vi "Cryostation Monitor and Control.vi"() -> ()   [LabVIEW 2020, in "instrument.Cryostation.lvclass"]
doc: "This VI will launch the Cryostation Instrument backend that will contunously monitor the state of the instrument and log to PGSQL."
uses:
  instrument.Cryostation/instrument.Cryostation.lvclass
  <userlib>/_OpenG.lib/appcontrol/appcontrol.llb/openg_application_control.lvlib
  <vilib>/JKI/JKI SMO/SMO/SMO.lvclass
  <vilib>/JKI/JKI SMO/SMO/Typedefs/SMOState --Enum.ctl
  <vilib>/JKI/JKI SMO/SMO.UI/SMO.UI.lvclass
  <userlib>/LevyLab/Instrument Framework/Instrument UI/Instrument UI.lvclass
  <userlib>/LevyLab/Instrument Framework/Instrument/Instrument.lvclass
  instrument.Cryostation UI/Instrument UI.Cryostation.lvclass
  C:/Program Files (x86)/National Instruments/LabVIEW 2020/user.lib/LevyLab/Instrument Framework/Instrument Types/Cryostat/Instrument.Cryostat.lvclass
  C:/Program Files (x86)/National Instruments/LabVIEW 2020/user.lib/LevyLab/Instrument Framework/Instrument/Instrument.lvclass
  C:/Program Files (x86)/National Instruments/LabVIEW 2020/vi.lib/JKI/JKI SMO/SMO/SMO.lvclass
  D:/Montana-Instruments-Cryostation/lvsrc/instrument.Cryostation/instrument.Cryostation.lvclass
  C:/Program Files (x86)/National Instruments/LabVIEW 2020/user.lib/LevyLab/Instrument Framework/Instrument UI/Instrument UI.lvclass
  C:/Program Files (x86)/National Instruments/LabVIEW 2020/vi.lib/JKI/JKI SMO/SMO.UI/SMO.UI.lvclass
  D:/Montana-Instruments-Cryostation/lvsrc/instrument.Cryostation UI/Instrument UI.Cryostation.lvclass
panel:
  out "version":string
  in  "Examine Configuration.ini":bool
  in  "Debug Mode":bool
  in  "Stop Application":bool caption="Stop"
  in  "Start Application":bool caption="Play"
  in  "Splash Status":string="Push Start to Start..." caption="String"
  out "UI SMO State":T1=enum."Stopped"
  out "SMO State":T1
  out "error out":errorcluster
  # "PPMS Monitor and Control.vi"
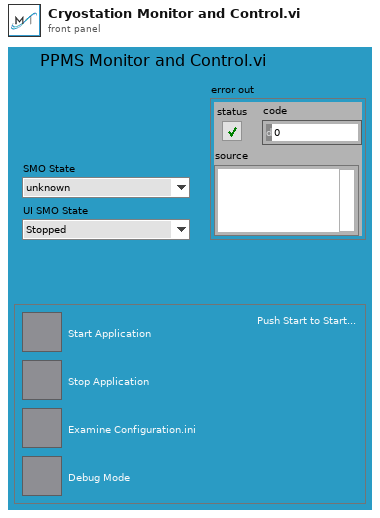
[diagram p1: front panel]
types:
  T1 = typedef "SMO.lvclass/SMOState --Enum.ctl" = enum16{"unknown", "Created", "Started", "Stopped"}
  T2 = enum32{"Invalid", "Standard", "Closed", "Hidden", "Minimized", "Maximized"}
  T3 = enum32{"invalid app kind", "Development System", "Run Time System", "Student Edition", "Embedded LabVIEW", "Evaluation", "Custom"}
  T4 = cluster{"Core":cluster{"Current VI Reference":refnum<vi>, "Close Panel on Exit?":bool}, "Instrument":refnum<class "instrument.Cryostation.lvclass">, "Instrument UI":refnum<class "Instrument UI.Cryostation.lvclass">}
  T5 = cluster{"Current VI Reference":refnum<vi>, "Close Panel on Exit?":bool}
  T6 = typedef "SMO.lvclass/Public Events.ctl" = cluster{"Error":refnum<user-event>, "State":refnum<user-event>, "Reserve State":refnum<user-event>}
  T7 = cluster{"Event Registration Refnum":refnum<event-registration>, "Event Registration Refnum":refnum<event-registration>}
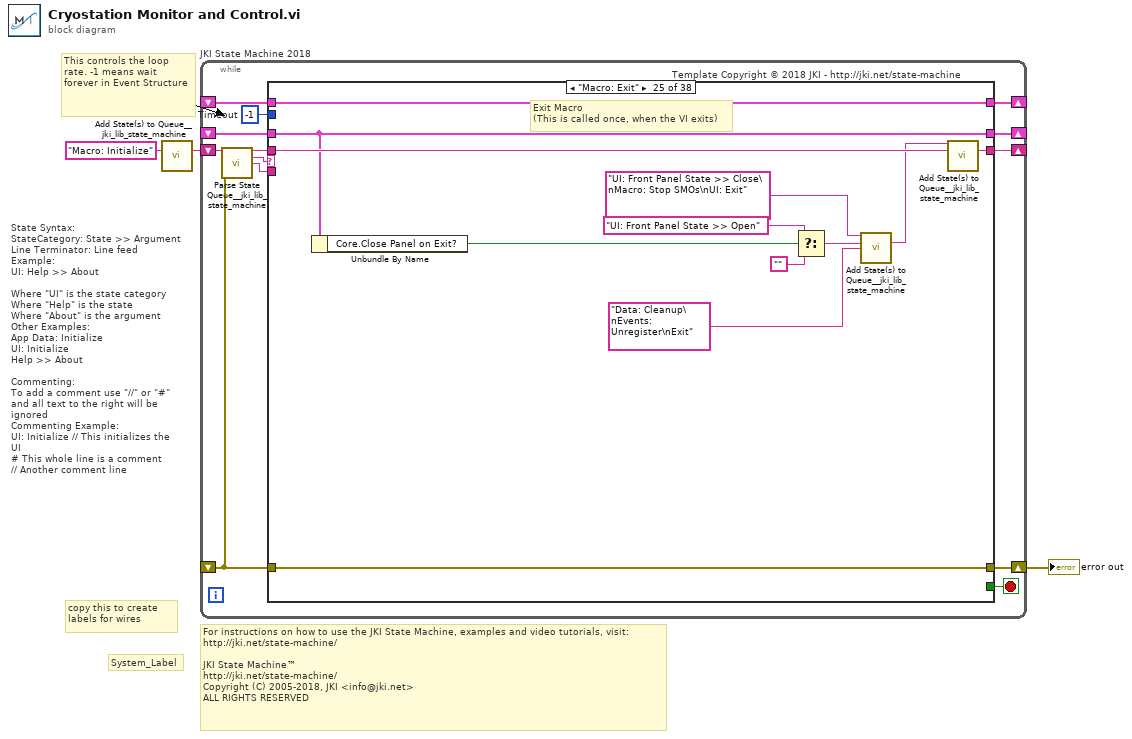
[diagram p0: block diagram]
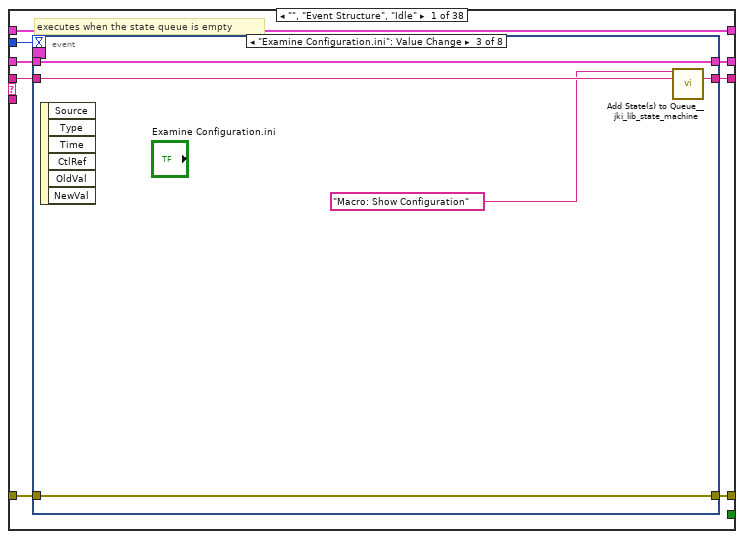
[diagram p2: hidden frame]
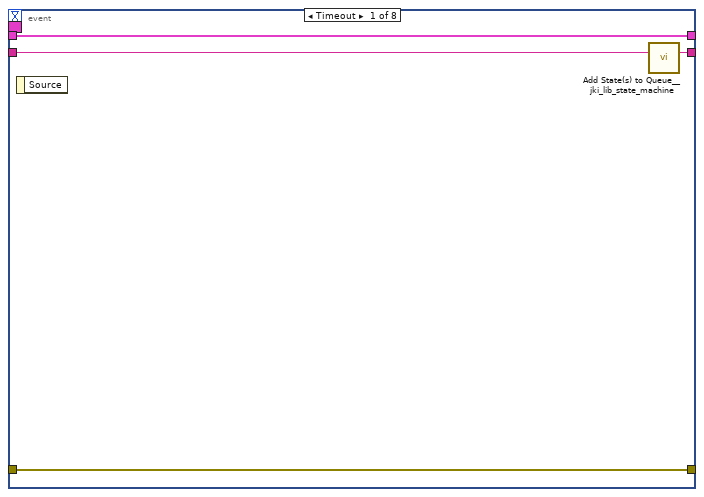
[diagram p3: hidden frame]
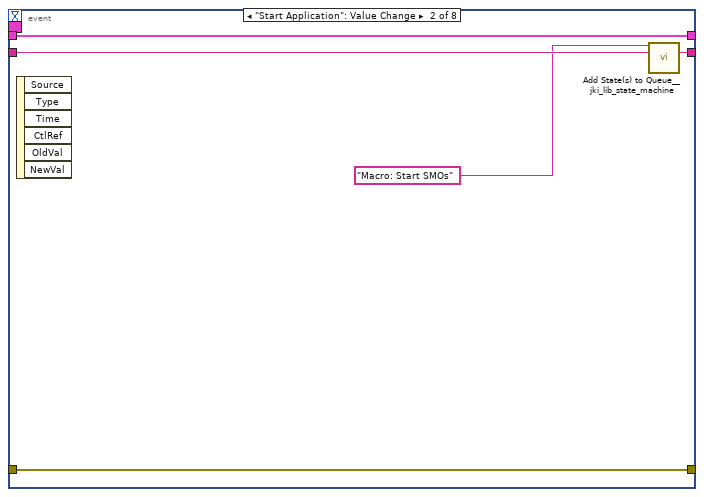
[diagram p4: hidden frame]
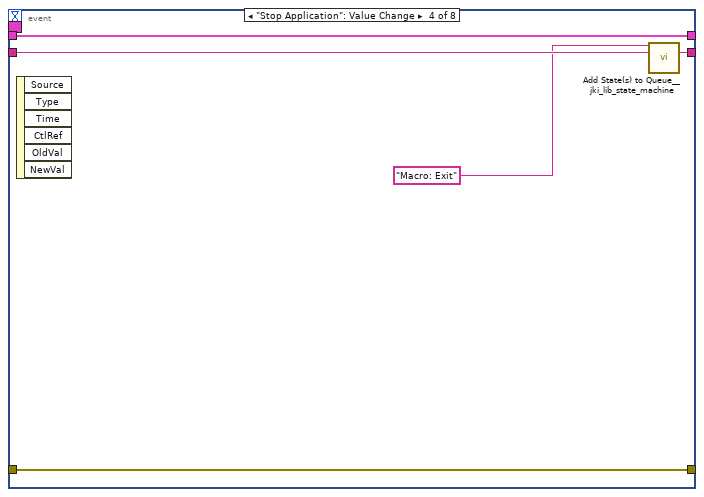
[diagram p5: hidden frame]
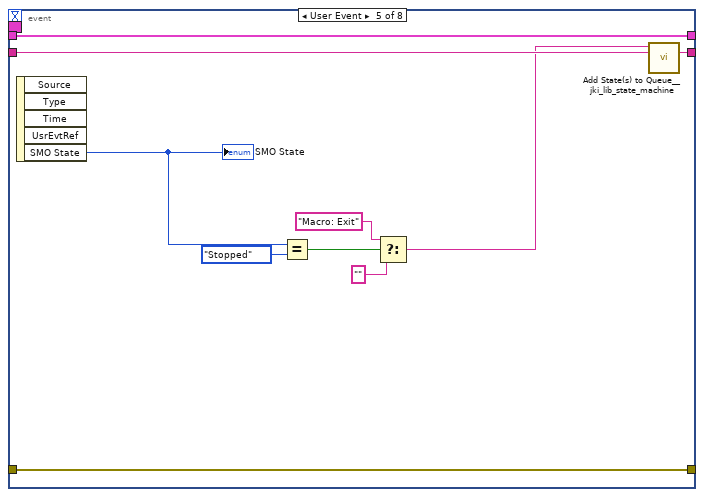
[diagram p6: hidden frame]
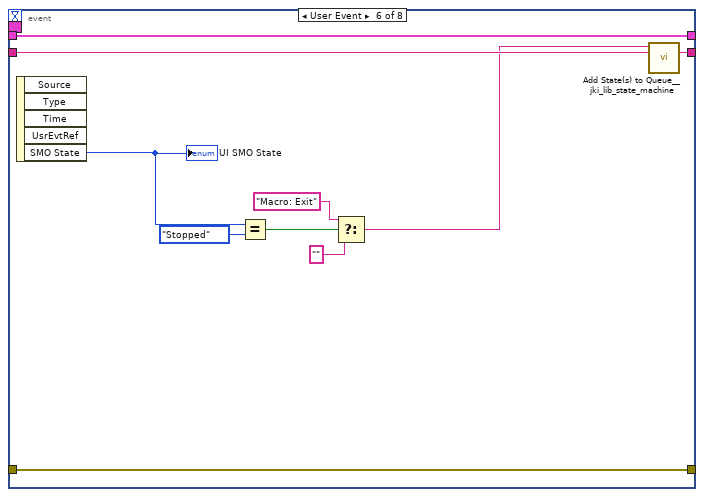
[diagram p7: hidden frame]
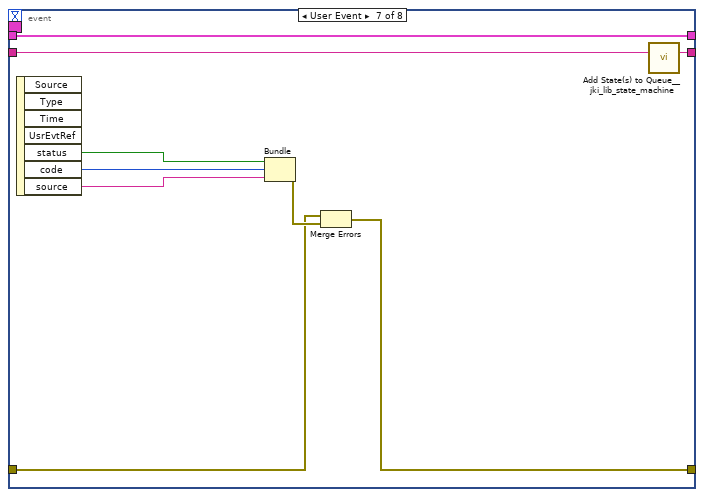
[diagram p8: hidden frame]
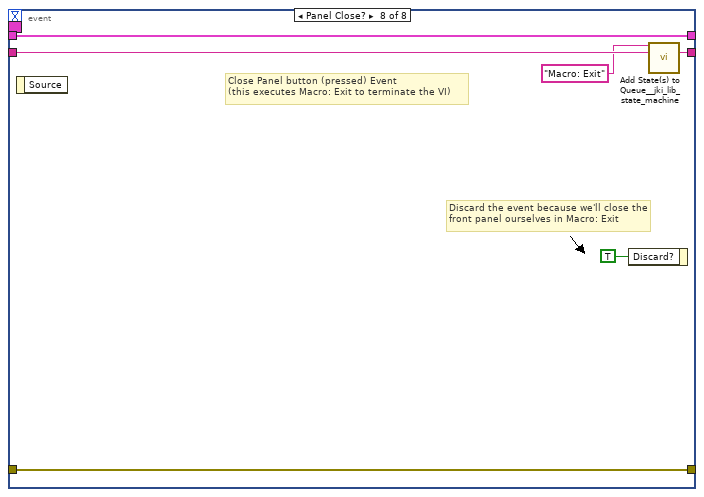
[diagram p9: hidden frame]
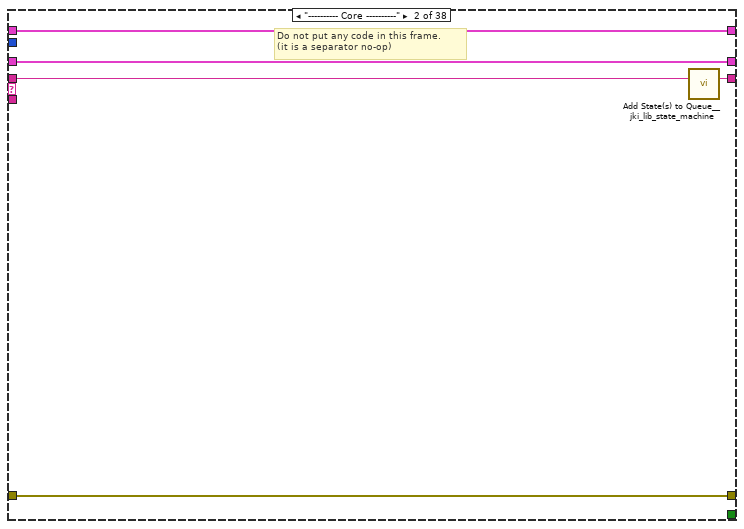
[diagram p10: hidden frame]
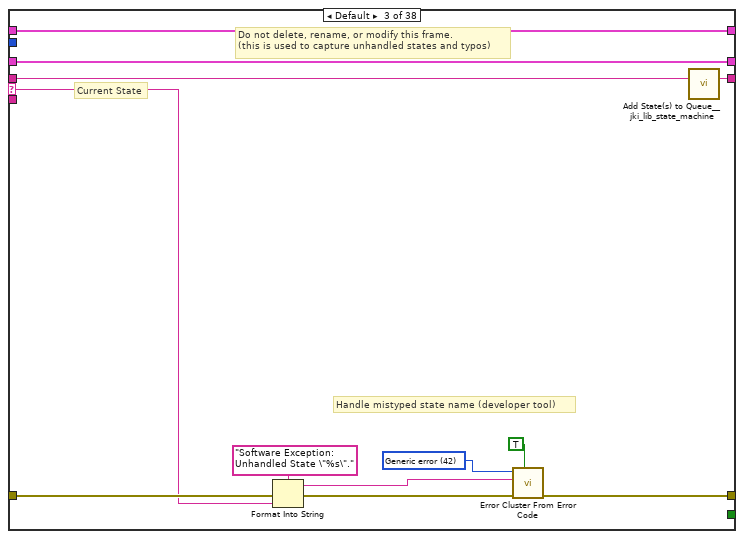
[diagram p11: hidden frame]
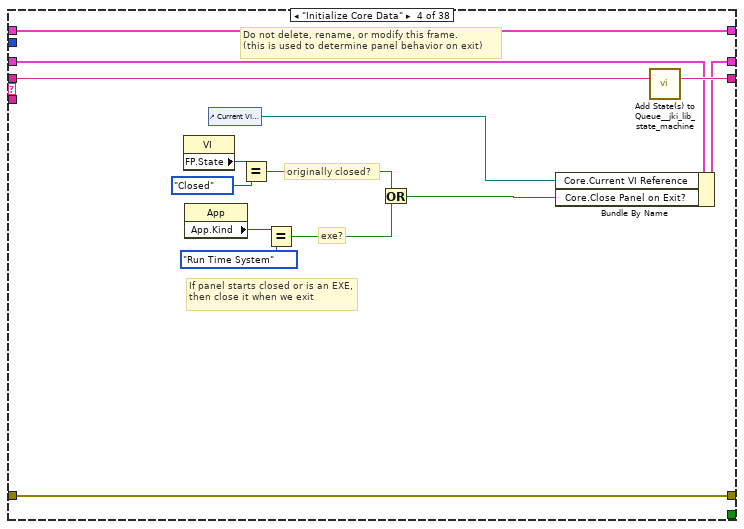
[diagram p12: hidden frame]
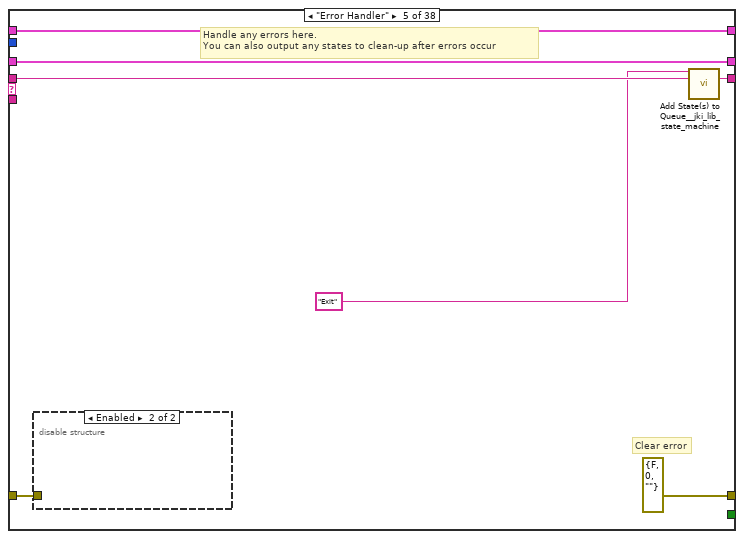
[diagram p13: hidden frame]
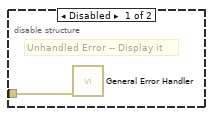
[diagram p14: hidden frame]
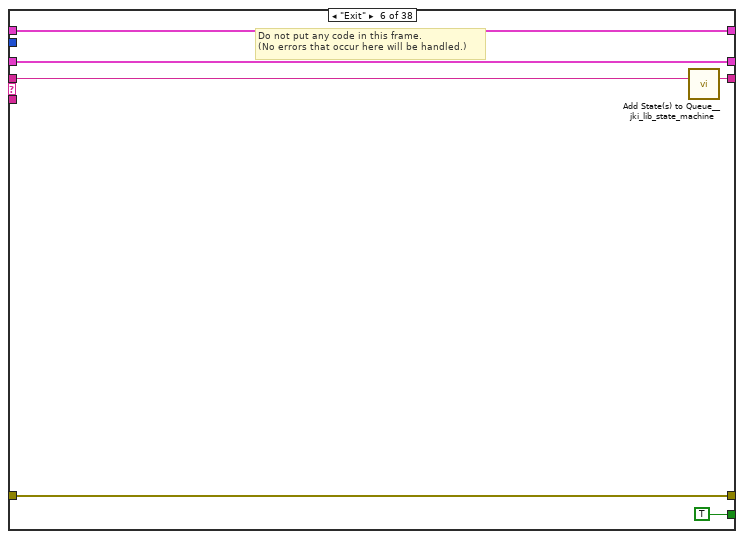
[diagram p15: hidden frame]
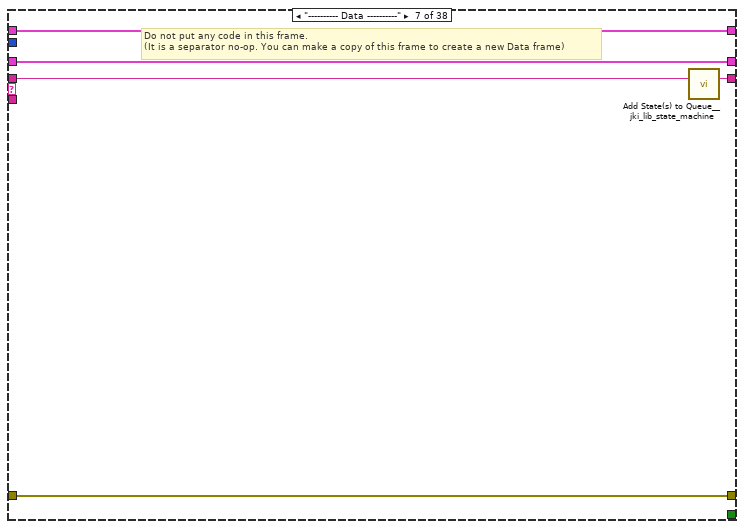
[diagram p16: hidden frame]
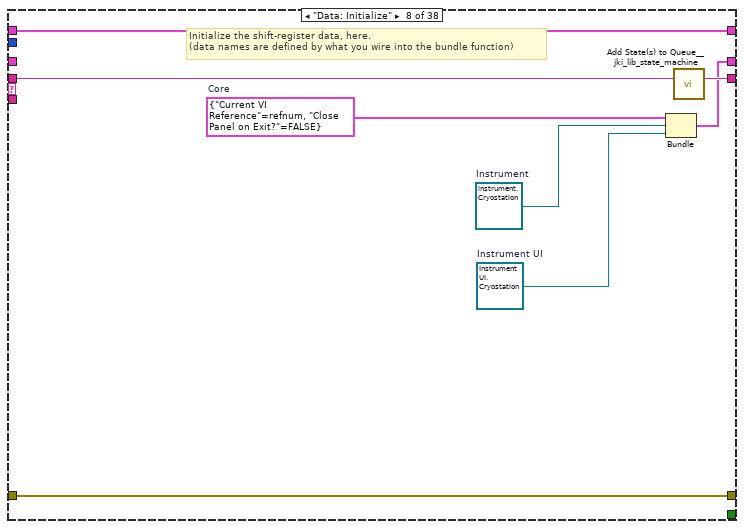
[diagram p17: hidden frame]
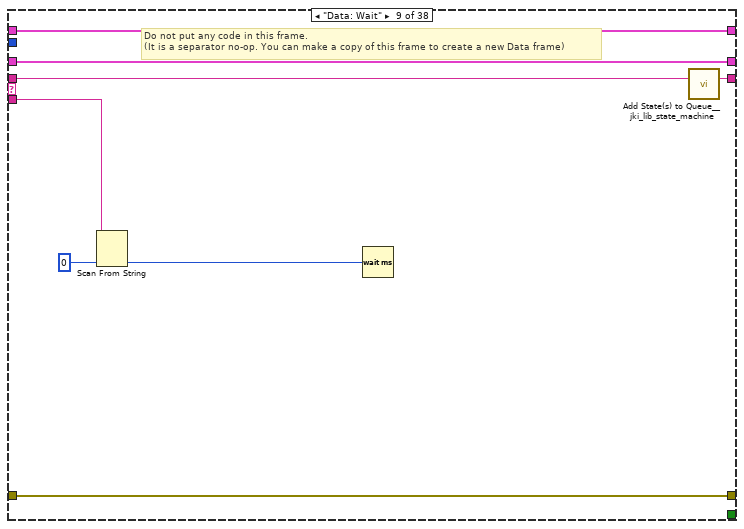
[diagram p18: hidden frame]
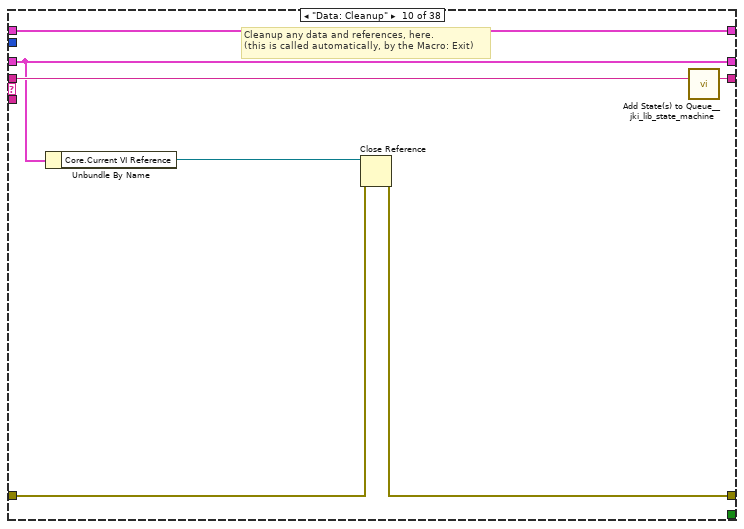
[diagram p19: hidden frame]
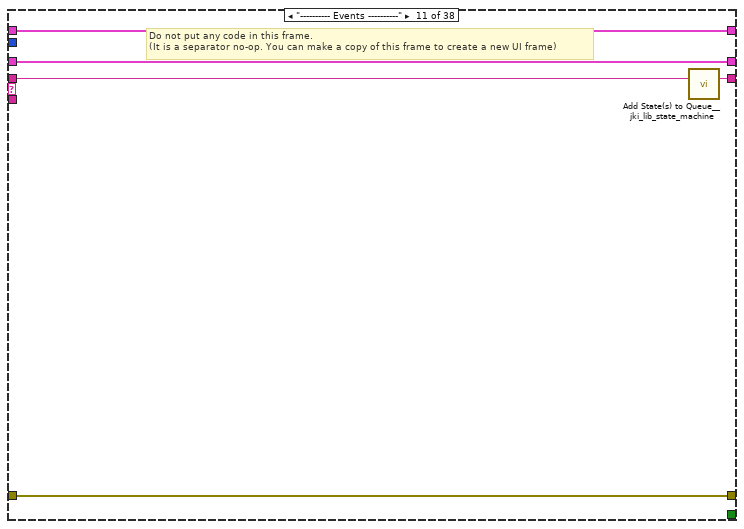
[diagram p20: hidden frame]
diagram:
  # "For instructions on how to use the JKI State Machine, examples and video tutorials, visit:\nhttp://jki.net/state-machine/\n\nJKI State Machine™\nhttp://jki.net/state-machine/\nCopyright (C) 2005-2018, JKI <info@jki.net>\nALL RIGHTS RESERVED"
  # "State Syntax:\nStateCategory: State >> Argument\nLine Terminator: Line feed\nExample:\nUI: Help >> About\n\nWhere \"UI\" is the state category\nWhere \"Help\" is the state\nWhere \"About\" is the argument\nOther Examples:\nApp Data: Initialize\nUI: Initialize\nHelp >> About\n\nCommenting:\nTo add a comment use \"//\" or \"#\" and all text to the right will be ignored\nCommenting Example:\nUI: Initialize // This initializes the UI\n# This whole line is a comment\n// Another comment line"
  # "copy this to create labels for wires"
  # "This controls the loop rate. -1 means wait forever in Event Structure"
  # "System_Label"
  n1 = call <vilib>:"Add State(s) to Queue__jki_lib_state_machine.vi"("State(s) in (\"\")"="Macro: Initialize") -> ("States Out"=w3:string)  [unwired: 14 in]
  n2 = while "JKI State Machine 2018" {
    shift-right: [w9] -> _
    shift-left: _ -> [w4]
    shift-right: [w12] -> w1
    shift-left: _ -> [w7]
    shift-right: [w11] -> _
    shift-left: w3 -> [w13]
    shift-right: [w6] -> _
    shift-left: _ -> [w5]
    stop <- w10 stop-if-true
    w8 = -1  # Timeout
    # "Template Copyright © 2018 JKI - http://jki.net/state-machine"
    n3 = call <vilib>:"Parse State Queue__jki_lib_state_machine.vi"("State Queue"=w13, "Error In (no error)"=w7) -> ("Remaining States"=w15:string, "Current State"=w16:string, "Arguments"=w14:string)  [unwired: 11 in]
    n4 = case shown="\"Macro: Exit\"" w16 {
      selector: w16 -> [_ _ w85 _ _ _ _ _ _ _ _ _ _ _ _ _ _ _ _ _ _ _ _ _ _ _ _ _ _ _ _ _ _ _ _ _ _ _]
      tunnel: w15 -> [w24 w83 w89 w109 w116 w123 w128 w136 w144 w151 w156 w169 w175 w180 w189 w196 w208 w282 w287 w292 w298 w304 w310 w316 w328 w333 w343 w352 w362 w369 w380 w395 w410 w425 w440 w449 w456 w461]
      tunnel: w14 -> [_ _ _ _ _ _ _ _ w137 _ _ _ _ _ _ w191 w202 _ _ _ _ _ _ _ _ _ _ _ _ _ _ _ _ _ _ _ w453 _]
      tunnel: [w21 w81 w91 w106 errorcluster {"status"=FALSE, "code"=0, "source"=""} ("error out") w120 w126 w133 w142 w147 w154 w158 w170 w178 w184 w192 w205 w278 w285 w290 w296 w302 w308 w314 w326 w331 w339 w344 w354 w363 w376 w391 w406 w422 w437 w447 w451 w459] -> w12
      tunnel: w7 -> [w20 w81 w90 w106 w112 w120 w126 w133 w142 w148 w154 w160 w171 w178 w186 w193 w206 w277 w285 w290 w296 w302 w308 w314 w326 w331 w340 w345 w355 w364 w373 w387 w403 w420 w433 w447 w452 w459]
      tunnel: [w23 w82 w88 w108 w115 w122 w127 w135 w143 w150 w155 w168 w174 w179 w188 w195 w207 w281 w286 w291 w297 w303 w309 w315 w327 w332 w342 w351 w361 w368 w379 w394 w409 w424 w439 w448 w455 w460] -> w11
      tunnel: [_ _ _ _ _ TRUE _ _ _ _ _ _ _ _ _ _ _ _ _ _ _ _ _ _ _ _ _ _ _ _ _ _ _ _ _ _ _ _] -> w10
      tunnel: [w19 w80 w87 w107 w113 w121 w125 w134 w141 w146 w153 w163 w173 w177 w187 w194 w204 w275 w284 w289 w295 w301 w307 w313 w325 w330 w338 w347 w356 w366 w377 w392 w407 w421 w436 w446 w454 w458] -> w9
      tunnel: w8 -> [w18 _ _ _ _ _ _ _ _ _ _ _ _ _ _ _ _ _ _ _ _ _ _ _ _ _ _ _ _ _ _ _ _ _ _ _ _ _]
      tunnel: [w17 w79 w84 w96 w110 w118 w124 w131 w140 w145 w152 w166 w172 w176 w185 w190 w201 w280 w283 w288 w293 w300 w306 w312 w319 w329 w341 w350 w360 w367 w378 w393 w408 w423 w438 w445 w450 w457] -> w6
      tunnel: w5 -> [w17 w79 w84 w96 w110 w118 w124 w131 w140 w145 w152 _ w172 w176 w185 w190 w201 w280 w283 w288 w293 w300 w306 w312 w319 w329 w341 w350 w360 w367 w378 w393 w408 w423 w438 w445 w450 w457]
      tunnel: w4 -> [w22 w80 w87 w102 w113 w121 w125 _ w141 w146 w153 w163 w173 w177 w187 w194 w204 w274 w284 w289 w295 w301 w307 w313 w325 w330 w335 w348 w357 w366 w377 w392 w407 w421 w436 w446 w454 w458]
      frame "", "Event Structure", "Idle" {
        # "executes when the state queue is empty"
        n5 = event shown="[2] \"Examine Configuration.ini\": Value Change" {
          selector: w17 -> [_ _ _ _ _ _ _ _]
          dyn-events: _ -> [_ _ _ _ _ _ _ _]
          timeout: w18 -> [_ _ _ _ _ _ _ _]
          tunnel: w24 -> [w28 w33 w38 w43 w53 w63 w72 w78]
          tunnel: [w27 w32 w37 w42 w52 w62 w71 w77] -> w23
          tunnel: w22 -> [w25 w30 w35 w40 w50 w60 w70 w75]
          tunnel: [w26 w31 w36 w41 w51 w61 w67 w76] -> w21
          tunnel: w20 -> [w26 w31 w36 w41 w51 w61 w68 w76]
          tunnel: [w25 w30 w35 w40 w50 w60 w70 w75] -> w19
          event Timeout {
            n6 = event-data() -> ()  [unwired: 1 in, 1 out]
            n7 = call <vilib>:"Add State(s) to Queue__jki_lib_state_machine.vi"("State(s) in (\"\")"=w28) -> ("States Out"=w27:string)  [unwired: 14 in]
          }
          event "Start Application": Value Change {
            n8 = event-data() -> ()  [unwired: 1 in, 6 out]
            n9 = call <vilib>:"Add State(s) to Queue__jki_lib_state_machine.vi"("State(s) in Front (\"\")"="Macro: Start SMOs" ("State(s) in Front (\"\")"), "State(s) in (\"\")"=w33) -> ("States Out"=w32:string)  [unwired: 13 in]
          }
          event "Examine Configuration.ini": Value Change {
            n10 = event-data() -> ()  [unwired: 1 in, 6 out]
            n11 = call <vilib>:"Add State(s) to Queue__jki_lib_state_machine.vi"("State(s) in Front (\"\")"="Macro: Show Configuration" ("State(s) in Front (\"\")"), "State(s) in (\"\")"=w38) -> ("States Out"=w37:string)  [unwired: 13 in]
          }
          event "Stop Application": Value Change {
            n12 = event-data() -> ()  [unwired: 1 in, 6 out]
            n13 = call <vilib>:"Add State(s) to Queue__jki_lib_state_machine.vi"("State(s) in Front (\"\")"="Macro: Exit" ("State(s) in Front (\"\")"), "State(s) in (\"\")"=w43) -> ("States Out"=w42:string)  [unwired: 13 in]
          }
          event User Event {
            n14 = event-data() -> ("SMO State"=w45:T1)  [unwired: 1 in, 4 out]
            "SMO State" <- w45
            n15 = Equal?(x=w45, y=SMOState_--Enum."Stopped") -> (x = y?=w48:bool)
            n16 = Select(t="Macro: Exit", s=w48, f="" ("State(s) in Front (\"\")")) -> (s? t:f=w44:string)
            n17 = call <vilib>:"Add State(s) to Queue__jki_lib_state_machine.vi"("State(s) in Front (\"\")"=w44, "State(s) in (\"\")"=w53) -> ("States Out"=w52:string)  [unwired: 13 in]
          }
          event User Event {
            n18 = event-data() -> ("SMO State"=w54:T1)  [unwired: 1 in, 4 out]
            "UI SMO State" <- w54
            n19 = Equal?(x=w54, y=SMOState_--Enum."Stopped") -> (x = y?=w58:bool)
            n20 = Select(t="Macro: Exit", s=w58, f="" ("State(s) in Front (\"\")")) -> (s? t:f=w56:string)
            n21 = call <vilib>:"Add State(s) to Queue__jki_lib_state_machine.vi"("State(s) in Front (\"\")"=w56, "State(s) in (\"\")"=w63) -> ("States Out"=w62:string)  [unwired: 13 in]
          }
          event User Event {
            n22 = event-data() -> ("status"=w64:bool, "code"=w66:i32, "source"=w65:string)  [unwired: 1 in, 4 out]
            n23 = Bundle("status"=w64, "code"=w66, "source"=w65) -> (w69:errorcluster)  [unwired: 1 in]
            n24 = Merge Errors(w68, w69) -> (w67:errorcluster)
            n25 = call <vilib>:"Add State(s) to Queue__jki_lib_state_machine.vi"("State(s) in (\"\")"=w72) -> ("States Out"=w71:string)  [unwired: 14 in]
          }
          event Panel Close? {
            # "Discard the event because we'll close the front panel ourselves in Macro: Exit"
            # "Close Panel button (pressed) Event\n(this executes Macro: Exit to terminate the VI)"
            n26 = event-data() -> ()  [unwired: 1 in, 1 out]
            n27 = event-data("Discard?"=TRUE) -> ()  [unwired: 1 in, 1 out]
            n28 = call <vilib>:"Add State(s) to Queue__jki_lib_state_machine.vi"("State(s) in Front (\"\")"="Macro: Exit", "State(s) in (\"\")"=w78) -> ("States Out"=w77:string)  [unwired: 13 in]
          }
        }
      }
      frame "---------- Core ----------" {
        # "Do not put any code in this frame.\n(it is a separator no-op)"
        n29 = call <vilib>:"Add State(s) to Queue__jki_lib_state_machine.vi"("State(s) in (\"\")"=w83) -> ("States Out"=w82:string)  [unwired: 14 in]
      }
      frame Default {
        w94 = 42 items=["No error", "Argument error", "Memory is full", "Out of zone", "End of file", "File already open", "Generic file I/O error", "File not found", "File permission error", "Disk is full", "Duplicate path", "Too many files open", "System feature not enabled", "Resource file not found", "Cannot add resource", "Resource not found", "Image not found", "Image memory error", "Pen does not exist", "Config type invalid", "Config token not found", "Config parse error", "Config memory error", "Bad external code format", "Bad external code offset", "External code not present", "Null window", "Destroy window error", "Null menu", "Print aborted", "Bad print record", "Print driver error", "Windows error during printing", "Memory error during printing", "Print dialog error", "Generic print error", "Invalid device refnum", "Device not found", "Device parameter error", "Device unit error", "Cannot open device", "Device call aborted", "Generic error", "Cancelled by user", "Object ID too low", "Object ID too high", "Object not in heap", "Unknown heap", "Unknown object (invalid DefProc)", "Unknown object (DefProc not in table)", "Message out of range", "Invalid (null) method", "Unknown message", "Manager call not supported", "Bad address", "Network operation in progress", "Network operation timed out", "Connection is busy", "Network attribute not supported", "Network error", "Address in use", "System out of memory", "Connection aborted", "Connection refused", "Not connected", "Already connected", "Connection closed", "Initialization error (interapplication manager)", "Bad occurrence", "Wait on unbound occurrence handler", "Occurrence queue overflow", "Datalog type conflict", "Unused", "Unrecognized type (interapplication manager)", "Memory corrupt", "Failed to make temporary DLL", "Old CIN version", "Drag socket not found", "Failed to load drop-object", "Failed to register OLE object", "Failed to release OLE object", "Format specifier type mismatch", "Unknown format specifier", "Too few format specifiers", "Too many format specifiers", "Scan failed", "Newer CIN version", "Error converting to variant", "Runtime menu error", "Password tampered", "Variant attribute not found", "Incompatible variant data type", "Event data is not available", "Event Store is not present", "Occurrence is not found", "Event Queue is not created", "Event info is not available", "Refnum passed is NULL", "Error retrieving Class GUID", "Error retrieving CoClass GUID", "Error retrieving TypeLib GUID.", "Bad built application magic bytes.", "Specific driver is different from the specific driver associated with the Logical Name.", "There is no session opened to the class driver.", "Max Error", "MAX - Error with config objects", "MAX - Error loading configuration", "MAX - Group not supported"]
        # "Current State"
        # "Do not delete, rename, or modify this frame.\n(this is used to capture unhandled states and typos)"
        # "Handle mistyped state name (developer tool)"
        n30 = Format Into String(format string="Software Exception: Unhandled State \"%s\"." ("message"), error in=w90, w85) -> (resulting string=w93:string, error out=w92:errorcluster)  [unwired: 1 in]
        n31 = call <vilib>:"Error Cluster From Error Code.vi"("show call chain? (False)"=TRUE, "error in (no error)"=w92, "error message (\"\")"=w93, "error code (0)"=w94) -> ("error out"=w91:errorcluster)  [unwired: 5 in]
        n32 = call <vilib>:"Add State(s) to Queue__jki_lib_state_machine.vi"("State(s) in (\"\")"=w89) -> ("States Out"=w88:string)  [unwired: 14 in]
      }
      frame "Initialize Core Data" {
        # "Do not delete, rename, or modify this frame.\n(this is used to determine panel behavior on exit)"
        # "originally closed?"
        # "exe?"
        # "If panel starts closed or is an EXE, then close it when we exit"
        n33 = property class="VI"() -> ("FP.State"=w99:T2)  [unwired: 2 in, 2 out]
        n34 = property class="App"() -> ("App.Kind"=w105:T3)  [unwired: 2 in, 2 out]
        n35 = control-ref of="Current VI Reference"() -> (w100:refnum<vi>)
        n36 = Equal?(x=w99, y=T2."Closed" ("Front Panel Window:State")) -> (x = y?=w97:bool)
        n37 = Equal?(x=w105, y=T3."Run Time System" ("Application:Kind")) -> (x = y?=w103:bool)
        n38 = Or(x=w97, y=w103) -> (x .or. y?=w101:bool)
        n39 = Bundle By Name(cluster=w102, "Core.Current VI Reference"=w100, "Core.Close Panel on Exit?"=w101) -> (w107:T4)
        n40 = call <vilib>:"Add State(s) to Queue__jki_lib_state_machine.vi"("State(s) in (\"\")"=w109) -> ("States Out"=w108:string)  [unwired: 14 in]
      }
      frame "Error Handler" {
        # "Handle any errors here.\nYou can also output any states to clean-up after errors occur"
        # "Clear error"
        n41 = disable-structure shown="Enabled" {
          disable-tunnel: w112 -> [w117 _]
          frame Disabled {
            # "Unhandled Error -- Display it"
            n42 = call <vilib>:"General Error Handler.vi"("error in (no error)"=w117) -> ()  [unwired: 10 in, 5 out]
          }
          frame Enabled {
          }
        }
        n43 = call <vilib>:"Add State(s) to Queue__jki_lib_state_machine.vi"("State(s) in Front (\"\")"="Exit", "State(s) in (\"\")"=w116) -> ("States Out"=w115:string)  [unwired: 13 in]
      }
      frame "Exit" {
        # "Do not put any code in this frame.\n(No errors that occur here will be handled.)"
        n44 = call <vilib>:"Add State(s) to Queue__jki_lib_state_machine.vi"("State(s) in (\"\")"=w123) -> ("States Out"=w122:string)  [unwired: 14 in]
      }
      frame "---------- Data ----------" {
        # "Do not put any code in this frame.\n(It is a separator no-op. You can make a copy of this frame to create a new Data frame)"
        n45 = call <vilib>:"Add State(s) to Queue__jki_lib_state_machine.vi"("State(s) in (\"\")"=w128) -> ("States Out"=w127:string)  [unwired: 14 in]
      }
      frame "Data: Initialize" {
        w130 = refnum<class "instrument.Cryostation.lvclass"> refnum  # Instrument
        w129 = refnum<class "Instrument UI.Cryostation.lvclass"> refnum  # Instrument UI
        w132 = T5 {"Current VI Reference"=refnum, "Close Panel on Exit?"=FALSE}  # Core
        # "Initialize the shift-register data, here.\n(data names are defined by what you wire into the bundle function)"
        n46 = Bundle("Core"=w132, "Instrument"=w130, "Instrument UI"=w129) -> (w134:T4)  [unwired: 1 in]
        n47 = call <vilib>:"Add State(s) to Queue__jki_lib_state_machine.vi"("State(s) in (\"\")"=w136) -> ("States Out"=w135:string)  [unwired: 14 in]
      }
      frame "Data: Wait" {
        # "Do not put any code in this frame.\n(It is a separator no-op. You can make a copy of this frame to create a new Data frame)"
        n48 = Scan From String(input string=w137, default 1=u32 0) -> (output 1=w138:u32)  [unwired: 3 in, 3 out]
        n49 = Wait (ms)(milliseconds to wait=w138) -> ()  [unwired: 1 out]
        n50 = call <vilib>:"Add State(s) to Queue__jki_lib_state_machine.vi"("State(s) in (\"\")"=w144) -> ("States Out"=w143:string)  [unwired: 14 in]
      }
      frame "Data: Cleanup" {
        # "Cleanup any data and references, here.\n(this is called automatically, by the Macro: Exit)"
        n51 = Unbundle By Name(w146) -> ("Core.Current VI Reference"=w149:refnum<vi>)
        n52 = Close Reference(reference=w149, error in (no error)=w148) -> (error out=w147:errorcluster)
        n53 = call <vilib>:"Add State(s) to Queue__jki_lib_state_machine.vi"("State(s) in (\"\")"=w151) -> ("States Out"=w150:string)  [unwired: 14 in]
      }
      frame "---------- Events ----------" {
        # "Do not put any code in this frame.\n(It is a separator no-op. You can make a copy of this frame to create a new UI frame)"
        n54 = call <vilib>:"Add State(s) to Queue__jki_lib_state_machine.vi"("State(s) in (\"\")"=w156) -> ("States Out"=w155:string)  [unwired: 14 in]
      }
      frame "Events: Register" {
        # "Do not put any code in this frame.\n(It is a separator no-op. You can make a copy of this frame to create a new UI frame)"
        n55 = Unbundle By Name(w163) -> ("Instrument"=w162:refnum<class "instrument.Cryostation.lvclass">, "Instrument UI"=w161:refnum<class "Instrument UI.Cryostation.lvclass">)
        n56 = call <vilib>:"GetPublicEvents.vi"("error in (no error)"=w160, "SMO"=w162) -> ("error out"=w159:errorcluster, "Public Events"=w164:T6)  [unwired: 7 in, 1 out]
        n57 = call <vilib>:"GetPublicEvents.vi"("error in (no error)"=w159, "SMO"=w161) -> ("error out"=w158:errorcluster, "Public Events"=w165:T6)  [unwired: 7 in, 1 out]
        n58 = register-events(w164) -> (reference out=w167:refnum<event-registration>)  [unwired: 2 in, 1 out]
        n59 = register-events(w165) -> (reference out=w157:refnum<event-registration>)  [unwired: 2 in, 1 out]
        n60 = Bundle("Event Registration Refnum"=w167, "Event Registration Refnum"=w157) -> (w166:T7)  [unwired: 1 in]
        n61 = call <vilib>:"Add State(s) to Queue__jki_lib_state_machine.vi"("State(s) in (\"\")"=w169) -> ("States Out"=w168:string)  [unwired: 14 in]
      }
      frame "Events: Unregister" {
        # "Do not put any code in this frame.\n(It is a separator no-op. You can make a copy of this frame to create a new UI frame)"
        n62 = Unregister For Events(event registration refnum=w172, error in=w171) -> (error out=w170:errorcluster)
        n63 = call <vilib>:"Add State(s) to Queue__jki_lib_state_machine.vi"("State(s) in (\"\")"=w175) -> ("States Out"=w174:string)  [unwired: 14 in]
      }
      frame "---------- UI ----------" {
        # "Do not put any code in this frame.\n(It is a separator no-op. You can make a copy of this frame to create a new UI frame)"
        n64 = call <vilib>:"Add State(s) to Queue__jki_lib_state_machine.vi"("State(s) in (\"\")"=w180) -> ("States Out"=w179:string)  [unwired: 14 in]
      }
      frame "UI: Initialize" {
        # "Initialize the User Interface, here.\n(this is called automatically, by the Macro: Init)"
        n65 = invoke on="Stop Application" class="Bool" method="Reinit To Default"() -> ()  [unwired: 3 in, 3 out]
        n66 = invoke on="error out" class="Clust (strict)" method="Reinit To Default"() -> ()  [unwired: 3 in, 3 out]
        n67 = invoke on="SMO State" class="Enum (strict)" method="Reinit To Default"() -> ()  [unwired: 3 in, 3 out]
        n68 = invoke on="Start Application" class="Bool" method="Reinit To Default"() -> ()  [unwired: 3 in, 3 out]
        n69 = call <userlib>:"Fit VI window to Largest Dec__ogtk.vi"("error in (no error)"=w186) -> ("error out"=w184:errorcluster)  [unwired: 5 in, 1 out]
        n70 = call <userlib>:"MGI Get Executable Version.vi"() -> ("Version"=w183:string)  [unwired: 7 in]
        n71 = Format Into String(format string="v%s", w183) -> (resulting string=→"version":string)  [unwired: 2 in, 1 out]
        n72 = call <vilib>:"Add State(s) to Queue__jki_lib_state_machine.vi"("State(s) in (\"\")"=w189) -> ("States Out"=w188:string)  [unwired: 14 in]
      }
      frame "UI: Cursor Set" {
        # "Argument"
        # "Set and Unset Cursor Busy.\n(Usage: \"UI: Cursor Set >> Busy|Idle\")"
        n73 = case shown="\"Idle\", Default" w191 {
          tunnel: w193 -> [w198 w200]
          tunnel: [w197 w199] -> w192
          frame "Idle", Default {
            n74 = call <vilib>:"Unset Busy.vi"("error in (no error)"=w198) -> ("error out"=w197:errorcluster)  [unwired: 10 in]
          }
          frame "Busy" {
            n75 = call <vilib>:"Set Busy.vi"("error in (no error)"=w200) -> ("error out"=w199:errorcluster)  [unwired: 9 in, 1 out]
          }
        }
        n76 = call <vilib>:"Add State(s) to Queue__jki_lib_state_machine.vi"("State(s) in (\"\")"=w196) -> ("States Out"=w195:string)  [unwired: 14 in]
      }
      frame "UI: Front Panel State" {
        # "Argument"
        # "Set Front Panel Open or Closed\n(Usage: \"UI: Front Panel State >> Open|Close\")"
        n77 = Unbundle By Name(w204) -> ("Core.Current VI Reference"=w203:refnum<vi>)
        n78 = case shown="\"Maximize\", \"Maximized\"" w202 {
          tunnel: w206 -> [w214 w229 w240 w253 w266]
          tunnel: [w216 w230 w242 w255 w268] -> w205
          tunnel: w203 -> [w215 w227 w241 w254 w267]
          frame "Open", "Standard", Default {
            w209 = T2."Standard" ("State")
            n79 = property class="VI"(reference=w215, error in=w214) -> (reference out=w212:refnum<vi>, error out=w213:errorcluster, "FP.State"=w211:T2)
            n80 = Not Equal?(x=w211, y=w209) -> (x != y?=w210:bool)
            n81 = case shown="True" w210 {
              tunnel: [w220 w222] -> w216
              tunnel: w213 -> [w219 w222]
              tunnel: w212 -> [w218 _]
              tunnel: w209 -> [w217 _]
              frame True {
                n82 = invoke class="VI" method="FP.Open"(reference=w218, error in=w219, "Activate"=TRUE, "State"=w217) -> (error out=w220:errorcluster)  [unwired: 1 in, 4 out]
              }
              frame False {
              }
            }
          }
          frame "Close", "Closed" {
            n83 = property class="VI"(reference=w227, error in=w229) -> (reference out=w226:refnum<vi>, error out=w228:errorcluster, "FP.State"=w224:T2)
            n84 = Not Equal?(x=w224, y=T2."Closed" ("Front Panel Window:State")) -> (x != y?=w223:bool)
            n85 = case shown="True" w223 {
              tunnel: [w231 w234] -> w230
              tunnel: w228 -> [w231 w233]
              tunnel: w226 -> [_ w232]
              frame False {
              }
              frame True {
                n86 = invoke class="VI" method="FP.Close"(reference=w232, error in=w233) -> (error out=w234:errorcluster)  [unwired: 1 in, 2 out]
              }
            }
          }
          frame "Hidden", "Hide" {
            w235 = T2."Hidden" ("State")
            n87 = property class="VI"(reference=w241, error in=w240) -> (reference out=w238:refnum<vi>, error out=w239:errorcluster, "FP.State"=w237:T2)
            n88 = Not Equal?(x=w237, y=w235) -> (x != y?=w236:bool)
            n89 = case shown="True" w236 {
              tunnel: [w246 w247] -> w242
              tunnel: w239 -> [w245 w247]
              tunnel: w238 -> [w244 _]
              tunnel: w235 -> [w243 _]
              frame True {
                n90 = invoke class="VI" method="FP.Open"(reference=w244, error in=w245, "State"=w243) -> (error out=w246:errorcluster)  [unwired: 2 in, 4 out]
              }
              frame False {
              }
            }
          }
          frame "Minimize", "Minimized" {
            w248 = T2."Minimized" ("State")
            n91 = property class="VI"(reference=w254, error in=w253) -> (reference out=w251:refnum<vi>, error out=w252:errorcluster, "FP.State"=w250:T2)
            n92 = Not Equal?(x=w250, y=w248) -> (x != y?=w249:bool)
            n93 = case shown="True" w249 {
              tunnel: [w259 w260] -> w255
              tunnel: w252 -> [w258 w260]
              tunnel: w251 -> [w257 _]
              tunnel: w248 -> [w256 _]
              frame True {
                n94 = invoke class="VI" method="FP.Open"(reference=w257, error in=w258, "State"=w256) -> (error out=w259:errorcluster)  [unwired: 2 in, 4 out]
              }
              frame False {
              }
            }
          }
          frame "Maximize", "Maximized" {
            w261 = T2."Maximized" ("State")
            n95 = property class="VI"(reference=w267, error in=w266) -> (reference out=w264:refnum<vi>, error out=w265:errorcluster, "FP.State"=w263:T2)
            n96 = Not Equal?(x=w263, y=w261) -> (x != y?=w262:bool)
            n97 = case shown="True" w262 {
              tunnel: [w272 w273] -> w268
              tunnel: w265 -> [w271 w273]
              tunnel: w264 -> [w270 _]
              tunnel: w261 -> [w269 _]
              frame True {
                n98 = invoke class="VI" method="FP.Open"(reference=w270, error in=w271, "State"=w269) -> (error out=w272:errorcluster)  [unwired: 2 in, 4 out]
              }
              frame False {
              }
            }
          }
        }
        n99 = call <vilib>:"Add State(s) to Queue__jki_lib_state_machine.vi"("State(s) in (\"\")"=w208) -> ("States Out"=w207:string)  [unwired: 14 in]
      }
      frame "UI: Open Configuration.ini" {
        # "Do not put any code in this frame.\n(It is a separator no-op. You can make a copy of this frame to create a new UI frame)"
        n100 = Unbundle By Name(w274) -> ("Instrument"=w279:refnum<class "instrument.Cryostation.lvclass">)
        n101 = call <userlib>:"Examine Configuration.vi"("error in (no error)"=w277, "Instrument in"=w279) -> ("error out"=w278:errorcluster, "Instrument out"=w276:refnum<class "instrument.Cryostation.lvclass">)  [unwired: 8 in]
        n102 = Bundle By Name(cluster=w274, "Instrument"=w276) -> (w275:T4)
        n103 = call <vilib>:"Add State(s) to Queue__jki_lib_state_machine.vi"("State(s) in (\"\")"=w282) -> ("States Out"=w281:string)  [unwired: 14 in]
      }
      frame "UI: Exit" {
        # "Do not put any code in this frame.\n(It is a separator no-op. You can make a copy of this frame to create a new UI frame)"
        n104 = invoke on="Start Application" class="Bool" method="Reinit To Default"() -> ()  [unwired: 3 in, 3 out]
        n105 = invoke on="Stop Application" class="Bool" method="Reinit To Default"() -> ()  [unwired: 3 in, 3 out]
        n106 = call <vilib>:"Add State(s) to Queue__jki_lib_state_machine.vi"("State(s) in (\"\")"=w287) -> ("States Out"=w286:string)  [unwired: 14 in]
      }
      frame "---------- Macro ----------" {
        # "Do not put any code in this frame.\n(It is a separator no-op. You can make a copy of this frame to create a new Macro frame)"
        n107 = call <vilib>:"Add State(s) to Queue__jki_lib_state_machine.vi"("State(s) in (\"\")"=w292) -> ("States Out"=w291:string)  [unwired: 14 in]
      }
      frame "Macro: Initialize" {
        # "Initialization Macro\n(This is called once, when the VI starts)"
        n108 = call <vilib>:"Add State(s) to Queue__jki_lib_state_machine.vi"("State(s) in Front (\"\")"="Data: Initialize\nInitialize Core Data\n//Events: Register\nUI: Initialize\nUI: Front Panel State >> Open\nSplash: Set Status >> Push Start to Start...", "State(s) in (\"\")"=w298) -> ("States Out"=w297:string)  [unwired: 13 in]
      }
      frame "Macro: Show Configuration" {
        # "Do not put any code in this frame.\n(It is a separator no-op. You can make a copy of this frame to create a new Macro frame)"
        n109 = call <vilib>:"Add State(s) to Queue__jki_lib_state_machine.vi"("State(s) in Front (\"\")"="Splash: Set Status >> Opening Configuration...\nUI: Open Configuration.ini\nData: Wait >> 1000\nSplash: Set Status >> ..." ("State(s) in Front (\"\")"), "State(s) in (\"\")"=w304) -> ("States Out"=w303:string)  [unwired: 13 in]
      }
      frame "Macro: Start SMOs" {
        # "Do not put any code in this frame.\n(It is a separator no-op. You can make a copy of this frame to create a new Macro frame)"
        n110 = call <vilib>:"Add State(s) to Queue__jki_lib_state_machine.vi"("State(s) in Front (\"\")"="Splash: Set Status >> Creating Instrument...\nSMO: Create Instrument\nData: Wait >> 100\nSplash: Set Status >> Creating Instrument UI...\nSMO: Create Instrument UI\nData: Wait >> 100\nSplash: Set Status >> Registering Events...\nEvents: Register\nData: Wait >> 100\nSplash: Set Status >> Starting Instrument...\nSMO: Start Instrument\nData: Wait >> 100\nSplash: Set Status >> Instrument Process Started...\nData: Wait >> 100\nSplash: Set Status >> Starting User Interface...\nSMO: Start Instrument UI\nData: Wait >> 100\nUI: Front Panel State >> Hide\nSMO: Show Instrument UI" ("State(s) in Front (\"\")"), "State(s) in (\"\")"=w310) -> ("States Out"=w309:string)  [unwired: 13 in]
      }
      frame "Macro: Stop SMOs" {
        # "Do not put any code in this frame.\n(It is a separator no-op. You can make a copy of this frame to create a new Macro frame)"
        n111 = call <vilib>:"Add State(s) to Queue__jki_lib_state_machine.vi"("State(s) in Front (\"\")"="UI: Front Panel State >> Show\nSplash: Set Status >> Stopping Instrument...\nSMO: Stop Instrument\nData: Wait >> 100\nSplash: Set Status >> Destroying Instrument...\nSMO: Destroy Instrument\nData: Wait >> 100\nSplash: Set Status >>Hiding UI...\nSMO: Hide Instrument UI\nData: Wait >> 100\nSplash: Set Status >> Stopping UI...\nSMO: Stop Instrument UI\nData: Wait >> 100\nSplash: Set Status >> Destroying UI...\nSMO: Destroy Instrument UI" ("State(s) in Front (\"\")"), "State(s) in (\"\")"=w316) -> ("States Out"=w315:string)  [unwired: 13 in]
      }
      frame "Macro: Exit" {
        # "Exit Macro\n(This is called once, when the VI exits)"
        n112 = Unbundle By Name(w325) -> ("Core.Close Panel on Exit?"=w324:bool)
        n113 = Select(t="UI: Front Panel State >> Open", s=w324, f="") -> (s? t:f=w321:string)
        n114 = call <vilib>:"Add State(s) to Queue__jki_lib_state_machine.vi"("State(s) in Front (\"\")"="UI: Front Panel State >> Close\nMacro: Stop SMOs\nUI: Exit", "State(s) in (\"\")"=w321, "State(s) at Back (\"\")"="Data: Cleanup\nEvents: Unregister\nExit") -> ("States Out"=w320:string)  [unwired: 12 in]
        n115 = call <vilib>:"Add State(s) to Queue__jki_lib_state_machine.vi"("State(s) in Front (\"\")"=w320, "State(s) in (\"\")"=w328) -> ("States Out"=w327:string)  [unwired: 13 in]
      }
      frame "---------- SMO ----------" {
        # "Do not put any code in this frame.\n(It is a separator no-op. You can make a copy of this frame to create a new Macro frame)"
        n116 = call <vilib>:"Add State(s) to Queue__jki_lib_state_machine.vi"("State(s) in (\"\")"=w333) -> ("States Out"=w332:string)  [unwired: 14 in]
      }
      frame "SMO: Create Instrument" {
        # "Do not put any code in this frame.\n(It is a separator no-op. You can make a copy of this frame to create a new Macro frame)"
        n117 = Unbundle By Name(w335) -> ("Instrument"=w334:refnum<class "instrument.Cryostation.lvclass">)
        n118 = call <userlib>:"Create Instrument SMO.vi"("error in (no error)"=w340, "Debug Mode? [F]"="Debug Mode", "Instrument in"=w334) -> ("error out"=w339:errorcluster, "Instrument out"=w337:refnum<class "instrument.Cryostation.lvclass">)  [unwired: 7 in]
        n119 = Bundle By Name(cluster=w335, "Instrument"=w337) -> (w338:T4)
        n120 = call <vilib>:"Add State(s) to Queue__jki_lib_state_machine.vi"("State(s) in (\"\")"=w343) -> ("States Out"=w342:string)  [unwired: 14 in]
      }
      frame "SMO: Start Instrument" {
        # "Do not put any code in this frame.\n(It is a separator no-op. You can make a copy of this frame to create a new Macro frame)"
        n121 = Unbundle By Name(w348) -> ("Instrument"=w349:refnum<class "instrument.Cryostation.lvclass">)
        n122 = call <vilib>:"Start.vi"("error in (no error)"=w345, "SMO"=w349) -> ("error out"=w344:errorcluster, "SMO out"=w346:refnum<class "instrument.Cryostation.lvclass">)  [unwired: 8 in]
        n123 = Bundle By Name(cluster=w348, "Instrument"=w346) -> (w347:T4)
        n124 = call <vilib>:"Add State(s) to Queue__jki_lib_state_machine.vi"("State(s) in (\"\")"=w352) -> ("States Out"=w351:string)  [unwired: 14 in]
      }
      frame "SMO: Create Instrument UI" {
        # "Do not put any code in this frame.\n(It is a separator no-op. You can make a copy of this frame to create a new Macro frame)"
        n125 = Unbundle By Name(w357) -> ("Instrument UI"=w353:refnum<class "Instrument UI.Cryostation.lvclass">, "Instrument"=w359:refnum<class "instrument.Cryostation.lvclass">)
        n126 = call <userlib>:"Create UI.vi"("error in (no error)"=w355, "Instrument in"=w359, "Instrument UI"=w353) -> ("error out"=w354:errorcluster, "Instrument UI out"=w358:refnum<class "Instrument UI.Cryostation.lvclass">)  [unwired: 7 in]
        n127 = Bundle By Name(cluster=w357, "Instrument UI"=w358) -> (w356:T4)
        n128 = call <vilib>:"Add State(s) to Queue__jki_lib_state_machine.vi"("State(s) in (\"\")"=w362) -> ("States Out"=w361:string)  [unwired: 14 in]
      }
      frame "SMO: Start Instrument UI" {
        # "Do not put any code in this frame.\n(It is a separator no-op. You can make a copy of this frame to create a new Macro frame)"
        n129 = Unbundle By Name(w366) -> ("Instrument UI"=w365:refnum<class "Instrument UI.Cryostation.lvclass">)
        n130 = call <vilib>:"Start.vi"("error in (no error)"=w364, "SMO"=w365) -> ("error out"=w363:errorcluster)  [unwired: 8 in, 1 out]
        n131 = call <vilib>:"Add State(s) to Queue__jki_lib_state_machine.vi"("State(s) in (\"\")"=w369) -> ("States Out"=w368:string)  [unwired: 14 in]
      }
      frame "SMO: Show Instrument UI" {
        # "Do not put any code in this frame.\n(It is a separator no-op. You can make a copy of this frame to create a new Macro frame)"
        n132 = Unbundle By Name(w377) -> ("Instrument UI"=w375:refnum<class "Instrument UI.Cryostation.lvclass">)
        n133 = call <vilib>:"GetState.vi"("error in (no error)"=w373, "SMO"=w375) -> ("error out"=w371:errorcluster, "SMO State"=w370:T1, "SMO out"=w374:refnum<class "Instrument UI.Cryostation.lvclass">)  [unwired: 7 in]
        n134 = call <vilib>:"Clear Errors.vi"("error in (no error)"=w371) -> ("error out"=w372:errorcluster)  [unwired: 5 in, 1 out]
        n135 = case shown="\"Started\"" w370 {
          tunnel: [w381 w384] -> w376
          tunnel: w374 -> [_ w383]
          tunnel: w372 -> [w381 w382]
          frame Default {
          }
          frame "Started" {
            n136 = call <vilib>:"Show.vi"("error in (no error)"=w382, "SMO.UI"=w383) -> ("error out"=w384:errorcluster)  [unwired: 8 in, 1 out]
          }
        }
        n137 = call <vilib>:"Add State(s) to Queue__jki_lib_state_machine.vi"("State(s) in (\"\")"=w380) -> ("States Out"=w379:string)  [unwired: 14 in]
      }
      frame "SMO: Destroy Instrument" {
        # "Do not put any code in this frame.\n(It is a separator no-op. You can make a copy of this frame to create a new Macro frame)"
        n138 = Unbundle By Name(w392) -> ("Instrument"=w390:refnum<class "instrument.Cryostation.lvclass">)
        n139 = call <vilib>:"GetState.vi"("error in (no error)"=w387, "SMO"=w390) -> ("error out"=w386:errorcluster, "SMO State"=w389:T1, "SMO out"=w385:refnum<class "instrument.Cryostation.lvclass">)  [unwired: 7 in]
        n140 = call <vilib>:"Clear Errors.vi"("error in (no error)"=w386) -> ("error out"=w388:errorcluster)  [unwired: 5 in, 1 out]
        n141 = case shown="\"Stopped\"" w389 {
          tunnel: [w396 w399] -> w391
          tunnel: w388 -> [w396 w398]
          tunnel: w385 -> [_ w397]
          frame Default {
          }
          frame "Stopped" {
            n142 = call <vilib>:"Destroy.vi"("error in (no error)"=w398, "SMO"=w397) -> ("error out"=w399:errorcluster)  [unwired: 9 in]
          }
        }
        n143 = call <vilib>:"Add State(s) to Queue__jki_lib_state_machine.vi"("State(s) in (\"\")"=w395) -> ("States Out"=w394:string)  [unwired: 14 in]
      }
      frame "SMO: Hide Instrument UI" {
        # "Do not put any code in this frame.\n(It is a separator no-op. You can make a copy of this frame to create a new Macro frame)"
        n144 = Unbundle By Name(w407) -> ("Instrument UI"=w405:refnum<class "Instrument UI.Cryostation.lvclass">)
        n145 = call <vilib>:"GetState.vi"("error in (no error)"=w403, "SMO"=w405) -> ("error out"=w401:errorcluster, "SMO State"=w400:T1, "SMO out"=w404:refnum<class "Instrument UI.Cryostation.lvclass">)  [unwired: 7 in]
        n146 = call <vilib>:"Clear Errors.vi"("error in (no error)"=w401) -> ("error out"=w402:errorcluster)  [unwired: 5 in, 1 out]
        n147 = case shown="Default" w400 {
          tunnel: [w411 w414] -> w406
          tunnel: w404 -> [_ w413]
          tunnel: w402 -> [w411 w412]
          frame Default {
          }
          frame "Started" {
            n148 = call <vilib>:"Hide.vi"("error in (no error)"=w412, "SMO.UI"=w413) -> ("error out"=w414:errorcluster)  [unwired: 8 in, 1 out]
          }
        }
        n149 = call <vilib>:"Add State(s) to Queue__jki_lib_state_machine.vi"("State(s) in (\"\")"=w410) -> ("States Out"=w409:string)  [unwired: 14 in]
      }
      frame "SMO: Stop Instrument UI" {
        # "Do not put any code in this frame.\n(It is a separator no-op. You can make a copy of this frame to create a new Macro frame)"
        n150 = Unbundle By Name(w421) -> ("Instrument UI"=w416:refnum<class "Instrument UI.Cryostation.lvclass">)
        n151 = call <vilib>:"GetState.vi"("error in (no error)"=w420, "SMO"=w416) -> ("error out"=w419:errorcluster, "SMO State"=w417:T1, "SMO out"=w415:refnum<class "Instrument UI.Cryostation.lvclass">)  [unwired: 7 in]
        n152 = call <vilib>:"Clear Errors.vi"("error in (no error)"=w419) -> ("error out"=w418:errorcluster)  [unwired: 5 in, 1 out]
        n153 = case shown="\"Created\", \"Started\"" w417 {
          tunnel: [w426 w429] -> w422
          tunnel: w415 -> [_ w428]
          tunnel: w418 -> [w426 w427]
          frame Default {
          }
          frame "Created", "Started" {
            n154 = call <vilib>:"Stop.vi"("error in (no error)"=w427, "SMO"=w428) -> ("error out"=w429:errorcluster)  [unwired: 8 in, 1 out]
          }
        }
        n155 = call <vilib>:"Add State(s) to Queue__jki_lib_state_machine.vi"("State(s) in (\"\")"=w425) -> ("States Out"=w424:string)  [unwired: 14 in]
      }
      frame "SMO: Destroy Instrument UI" {
        # "Do not put any code in this frame.\n(It is a separator no-op. You can make a copy of this frame to create a new Macro frame)"
        n156 = Unbundle By Name(w436) -> ("Instrument UI"=w435:refnum<class "Instrument UI.Cryostation.lvclass">)
        n157 = call <vilib>:"GetState.vi"("error in (no error)"=w433, "SMO"=w435) -> ("error out"=w432:errorcluster, "SMO State"=w430:T1, "SMO out"=w434:refnum<class "Instrument UI.Cryostation.lvclass">)  [unwired: 7 in]
        n158 = call <vilib>:"Clear Errors.vi"("error in (no error)"=w432) -> ("error out"=w431:errorcluster)  [unwired: 5 in, 1 out]
        n159 = case shown="Default" w430 {
          tunnel: w431 -> [w441 w444]
          tunnel: [w441 w443] -> w437
          tunnel: w434 -> [_ w442]
          frame Default {
          }
          frame "Stopped" {
            n160 = call <vilib>:"Destroy.vi"("error in (no error)"=w444, "SMO"=w442) -> ("error out"=w443:errorcluster)  [unwired: 9 in]
          }
        }
        n161 = call <vilib>:"Add State(s) to Queue__jki_lib_state_machine.vi"("State(s) in (\"\")"=w440) -> ("States Out"=w439:string)  [unwired: 14 in]
      }
      frame "---------- Splash ----------" {
        # "Template Separator\n(You can make a copy of, or modify, this frame)"
        n162 = call <vilib>:"Add State(s) to Queue__jki_lib_state_machine.vi"("State(s) in (\"\")"=w449) -> ("States Out"=w448:string)  [unwired: 14 in]
      }
      frame "Splash: Set Status" {
        # "Your code here.\n(You can make a copy of, or modify, this frame)"
        n163 = property on="Splash Status" class="Str"(error in=w452, "Value"=w453) -> (error out=w451:errorcluster)  [unwired: 1 in, 1 out]
        n164 = call <vilib>:"Add State(s) to Queue__jki_lib_state_machine.vi"("State(s) in (\"\")"=w456) -> ("States Out"=w455:string)  [unwired: 14 in]
      }
      frame "Splash: 2" {
        # "Your code here.\n(You can make a copy of, or modify, this frame)"
        n165 = call <vilib>:"Add State(s) to Queue__jki_lib_state_machine.vi"("State(s) in (\"\")"=w461) -> ("States Out"=w460:string)  [unwired: 14 in]
      }
    }
  }
  "error out" <- w1
